vi "XLP80_GUI_CVM.vi"(8 "err in":errorcluster) -> (0 "err out":errorcluster)   [LabVIEW 2021]
uses:
  XLP80_General_Libs/WL_Libs_V14.25/WL_TypeDefs_V14.00.llb/WL_TypeDefs_EnumState.ctl
  XLP80_ProjectLibs/FCE_TS_SMART_V001.llb/XLP80_SMART_GUIGlobals.vi
  XLP80_General_Libs/WL_Libs_V14.25/WL_Frontpanel_V14.01.llb/WL_Frontpanel_GblStatus.vi
  XLP80_ProjectLibs/FCE_TS_SMART_V001.llb/FCE_TS_SMART_Globals.vi
panel:
  out "CVM_Digital_horizontal":sgl[](array[numeric]) format="%03.0f"
  in  "but_Close":bool
  out "Total  Voltage":dbl format="%.0f mV"
  out "Lowest Cell Voltage":dbl format="%.0f mV"
  out "Highest Cell Voltage":dbl format="%.0f mV"
  out "CVM_CellNo_vertical":i32[](array[numeric]) format="%0.0f"
  out "CVM_Digital_vertical":sgl[](array[numeric]) format="%0.0f"
  out "CVM":sgl[][](graph)
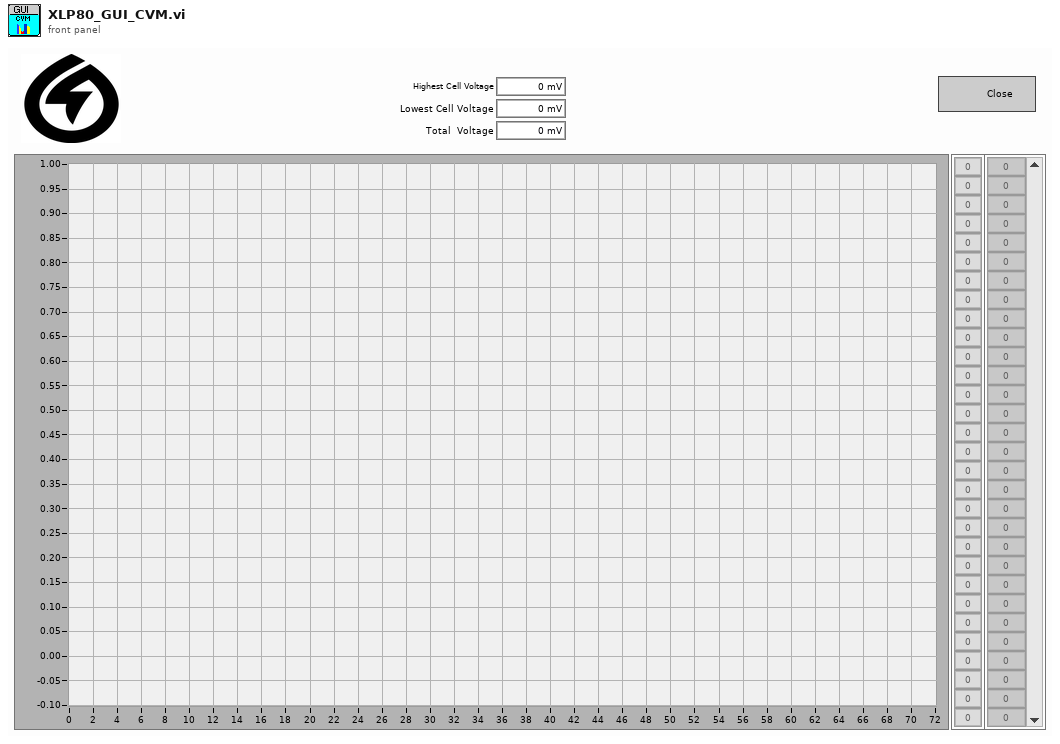
[diagram p1: front panel]
types:
  T1 = enum32{"Invalid", "Standard", "Closed", "Hidden", "Minimized", "Maximized"}
  T2 = typedef "WL_TypeDefs_EnumState.ctl" = enum16{"Init", "Run", "End"}
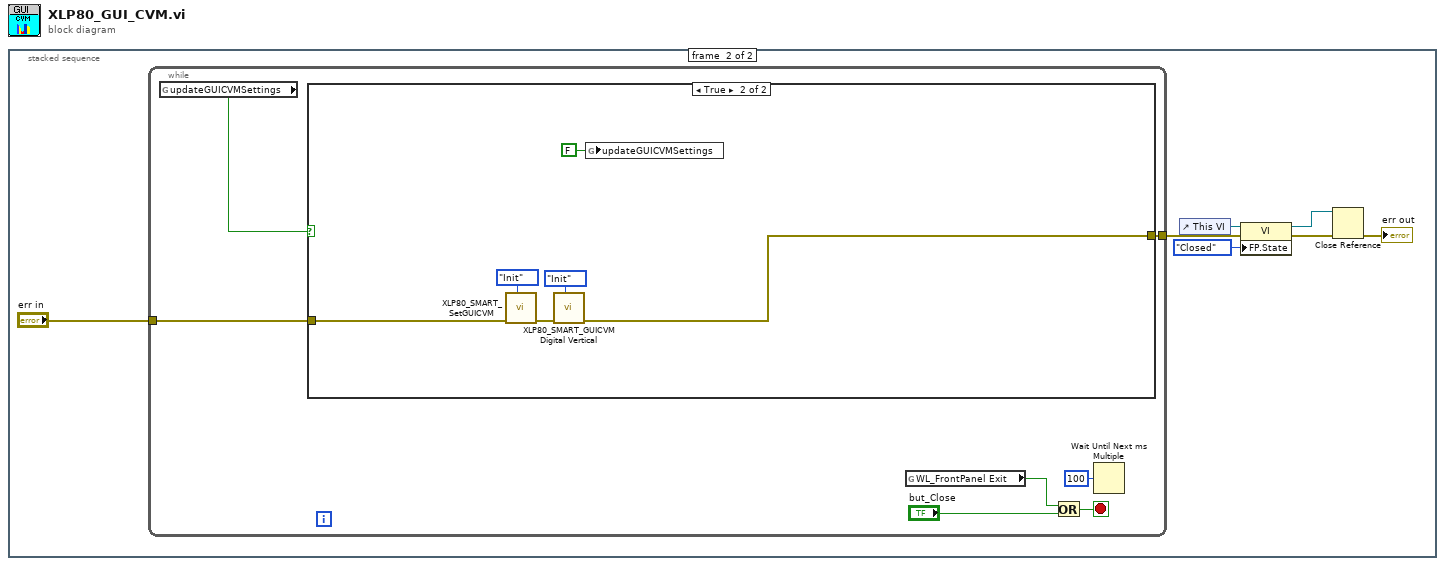
[diagram p0: block diagram]
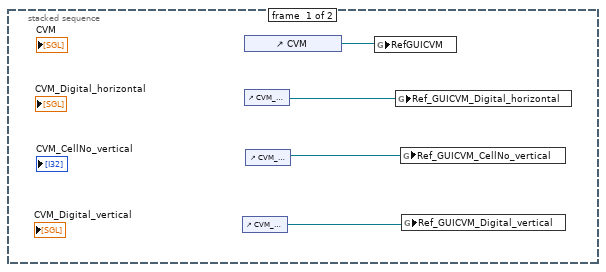
[diagram p2: hidden frame]
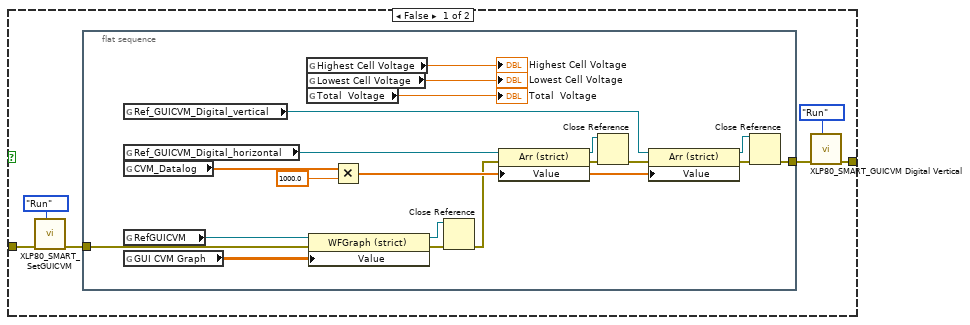
[diagram p3: hidden frame]
diagram:
  n1 = stacked-sequence {
    frame #0 {
      n2 = control-ref of="CVM_Digital_vertical"() -> (w1:refnum<vi>)
      n3 = control-ref of="CVM"() -> (w4:refnum<vi>)
      n4 = control-ref of="CVM_Digital_horizontal"() -> (w3:refnum<vi>)
      n5 = control-ref of="CVM_CellNo_vertical"() -> (w2:refnum<vi>)
      n6 = global write "XLP80_SMART_GUIGlobals.vi" "RefGUICVM"(w4) -> ()
      n7 = global write "XLP80_SMART_GUIGlobals.vi" "Ref_GUICVM_Digital_horizontal"(w3) -> ()
      n8 = global write "XLP80_SMART_GUIGlobals.vi" "Ref_GUICVM_CellNo_vertical"(w2) -> ()
      n9 = global write "XLP80_SMART_GUIGlobals.vi" "Ref_GUICVM_Digital_vertical"(w1) -> ()
    }
    frame #1 {
      n10 = while {
        tunnel: "err in" -> [w14]
        tunnel: [w13] -> w11
        stop <- w17 stop-if-true
        n11 = global read "XLP80_SMART_GUIGlobals.vi" "updateGUICVMSettings"() -> (w12:bool)
        n12 = case shown="True" w12 {
          tunnel: w14 -> [w23 w48]
          tunnel: [w20 w46] -> w13
          frame False {
            n13 = call "XLP80_SMART_SetGUICVM.vi"("State"=WL_TypeDefs_EnumState."Run", "err in"=w23) -> ("err out"=w22:errorcluster)  [unwired: 9 in]
            n14 = flat-sequence {
              tunnel: [w37] -> w21
              tunnel: w22 -> [w32]
              frame #0 {
                n15 = global read "XLP80_SMART_GUIGlobals.vi" "Ref_GUICVM_Digital_vertical"() -> (w28:refnum<vi>)
                n16 = global read "XLP80_SMART_GUIGlobals.vi" "Ref_GUICVM_Digital_horizontal"() -> (w29:refnum<vi>)
                n17 = global read "FCE_TS_SMART_Globals.vi" "CVM_Datalog"() -> (w33:sgl[])
                n18 = global read "XLP80_SMART_GUIGlobals.vi" "RefGUICVM"() -> (w31:refnum<vi>)
                n19 = global read "XLP80_SMART_GUIGlobals.vi" "GUI CVM Graph"() -> (w30:sgl[][])
                n20 = global read "XLP80_SMART_GUIGlobals.vi" "Highest Cell Voltage"() -> (→"Highest Cell Voltage":dbl)
                n21 = global read "XLP80_SMART_GUIGlobals.vi" "Lowest Cell Voltage"() -> (→"Lowest Cell Voltage":dbl)
                n22 = global read "XLP80_SMART_GUIGlobals.vi" "Total  Voltage"() -> (→"Total  Voltage":dbl)
                n23 = property class="WFGraph (strict)"(reference=w31, error in=w32, "Value"=w30) -> (reference out=w38:refnum<vi>, error out=w44:errorcluster)
                n24 = Multiply(x=w33, y=sgl 1000.0 ("Numeric")) -> (x*y=w41:sgl[])
                n25 = Close Reference(reference=w38, error in (no error)=w44) -> (error out=w39:errorcluster)
                n26 = property class="Arr (strict)"(reference=w29, error in=w39, "Value"=w41) -> (reference out=w34:refnum<vi>, error out=w42:errorcluster)
                n27 = Close Reference(reference=w34, error in (no error)=w42) -> (error out=w35:errorcluster)
                n28 = property class="Arr (strict)"(reference=w28, error in=w35, "Value"=w41) -> (reference out=w36:refnum<vi>, error out=w40:errorcluster)
                n29 = Close Reference(reference=w36, error in (no error)=w40) -> (error out=w37:errorcluster)
              }
            }
            n30 = call "XLP80_SMART_GUICVM Digital Vertical.vi"("CVM"=enum16{"Init", "Run"}."Run", "err in"=w21) -> ("err out"=w20:errorcluster)  [unwired: 9 in]
          }
          frame True {
            n31 = call "XLP80_SMART_SetGUICVM.vi"("State"=WL_TypeDefs_EnumState."Init", "err in"=w48) -> ("err out"=w47:errorcluster)  [unwired: 9 in]
            n32 = call "XLP80_SMART_GUICVM Digital Vertical.vi"("CVM"=enum16{"Init", "Run"}."Init", "err in"=w47) -> ("err out"=w46:errorcluster)  [unwired: 9 in]
            n33 = global write "XLP80_SMART_GUIGlobals.vi" "updateGUICVMSettings"(FALSE ("updateGUICVMSettings")) -> ()
          }
        }
        n34 = global read "WL_Frontpanel_GblStatus.vi" "WL_FrontPanel Exit"() -> (w15:bool)
        n35 = Or(x=w15, y="but_Close") -> (x .or. y?=w17:bool)
        n36 = Wait Until Next ms Multiple(millisecond multiple=u32 100) -> ()  [unwired: 1 out]
      }
      n37 = control-ref of="This VI"() -> (w9:refnum<vi>)
      n38 = property class="VI"(reference=w9, error in=w11, "FP.State"=T1."Closed" ("Front Panel Window:State")) -> (reference out=w6:refnum<vi>, error out=w10:errorcluster)
      n39 = Close Reference(reference=w6, error in (no error)=w10) -> (error out=→"err out":errorcluster)
    }
  }
